vi "Calculate frame period.vi"(9 "Dwell time (us)":dbl=0.01, 10 "AOD fill time (us)":dbl=24.4, 11 "Frame size (pixels in single dimension)":i32=512) -> (3 "Frame period (ms)":dbl)   [LabVIEW 2013]
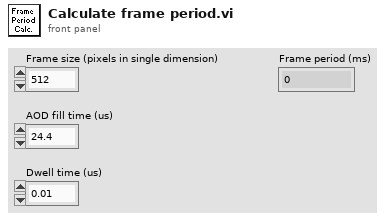
[diagram p1: front panel]
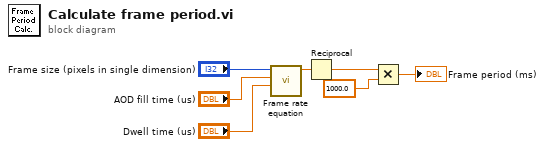
[diagram p0: block diagram]
diagram:
  n1 = call "Frame rate equation.vi"("Dwell time (us)"="Dwell time (us)", "AOD fill time (us)"="AOD fill time (us)", "Frame size (single dimension)"="Frame size (pixels in single dimension)") -> ("FrameRate (fps)"=w2:dbl)  [unwired: 8 in]
  n2 = Reciprocal(x=w2) -> (1/x=w3:dbl)
  n3 = Multiply(x=w3, y=1000.0) -> (x*y=→"Frame period (ms)":dbl)
